vi "ReceiveGetAnalogCommand.vi"(8 "entrée d'erreur (pas d'erreur)":errorcluster, 11 "Connexion réseau UDP en entrée":refnum<k16>) -> (0 "sortie d'erreur":errorcluster, 1 "Connexion réseau UDP en sortie":refnum<k16>, 2 "Response Command":u8[](array[numeric]), 3 "Numérique":u16)   [LabVIEW 2021]
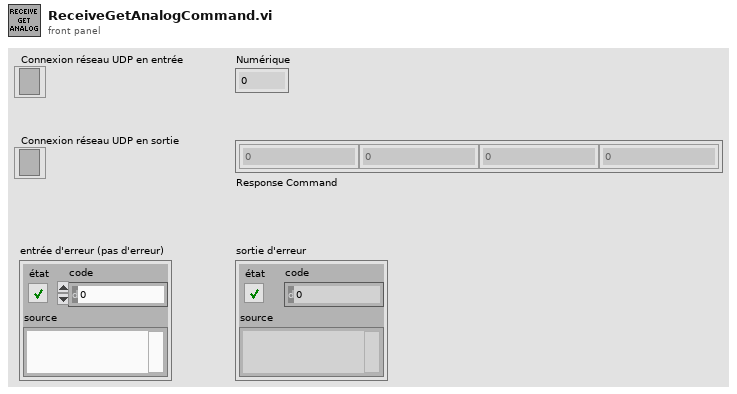
[diagram p1: front panel]
types:
  T1 = typedef "CommandType.ctl" = u8[]
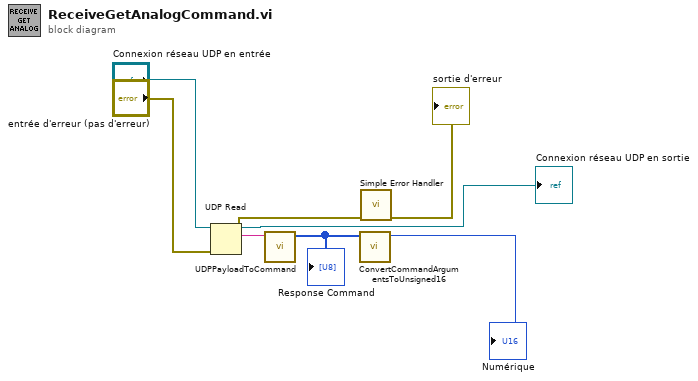
[diagram p0: block diagram]
diagram:
  n1 = UDP Read(connection ID="Connexion réseau UDP en entrée", 8:"entrée d'erreur (pas d'erreur)") -> (data out=w2:string, error out=w3:errorcluster, 3:→"Connexion réseau UDP en sortie":refnum<k16>)  [unwired: 2 in, 2 out]
  n2 = call "UDPPayloadToCommand.vi"("UDP Payload"=w2) -> ("Command"=w8:T1)  [unwired: 10 in]
  "Response Command" <- w8
  n3 = call "ConvertCommandArgumentsToUnsigned16.vi"("Command"=w8) -> ("Numérique"=→"Numérique":u16)  [unwired: 10 in]
  n4 = call <vilib>:"Simple Error Handler.vi"("error in (no error)"=w3) -> ("error out"=→"sortie d'erreur":errorcluster)  [unwired: 4 in, 4 out]
